vi "make_axes_labels_number_axis.vi"(0 "Merged Array Out":T3(array[cluster]), 1 "View Direction":T1(ring), 2 "Which Axis?":T2(ring)=enum."Z Opposite", 3 "Draw Y?":bool, 5 "from":dbl, 9 "to":dbl, 11 "axis-offset":dbl, 12 "Font Color":u32(colorbox)=4863, 14 "Font Size":dbl min=-1.7976931348623157e+308 max=1.7976931348623157e+308) -> (4 "Scene:New Object":refnum<vi>, 6 "Max Width":dbl)   [LabVIEW 2020, in "3DPC_SurfacePlot.xctl"]
uses:
  <vilib>/Native 3D Graph/xcontrol/3DPC_SurfacePlot.xctl
  <vilib>/Utility/miscctls.llb/LV3DPointTypeDef.ctl
panel:
  in  "Antialiasing":bool
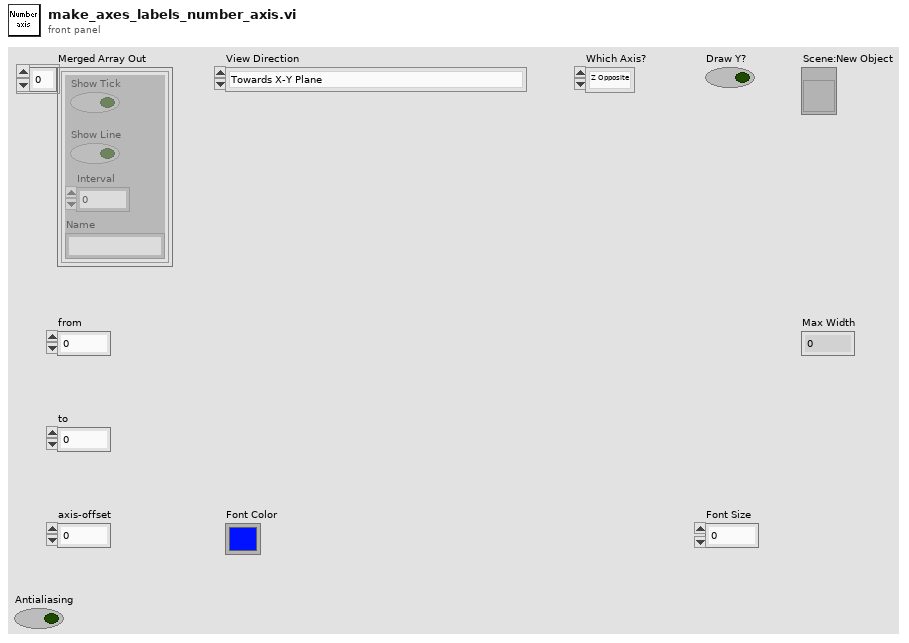
[diagram p1: front panel]
types:
  T1 = enum32{"Towards X-Y Plane", "Towards Y-Z Plane", "Towards X-Z Plane", "User Define"}
  T2 = enum16{"X", "Y", "Z", "X Opposite", "Y Opposite", "Z Opposite"}
  T3 = cluster{"Show Tick":bool, "Show Line":bool, "Interval":sgl, "Name":string}[]
  T4 = typedef "LV3DPointTypeDef.ctl" = cluster{"X":sgl, "Y":sgl, "Z":sgl}
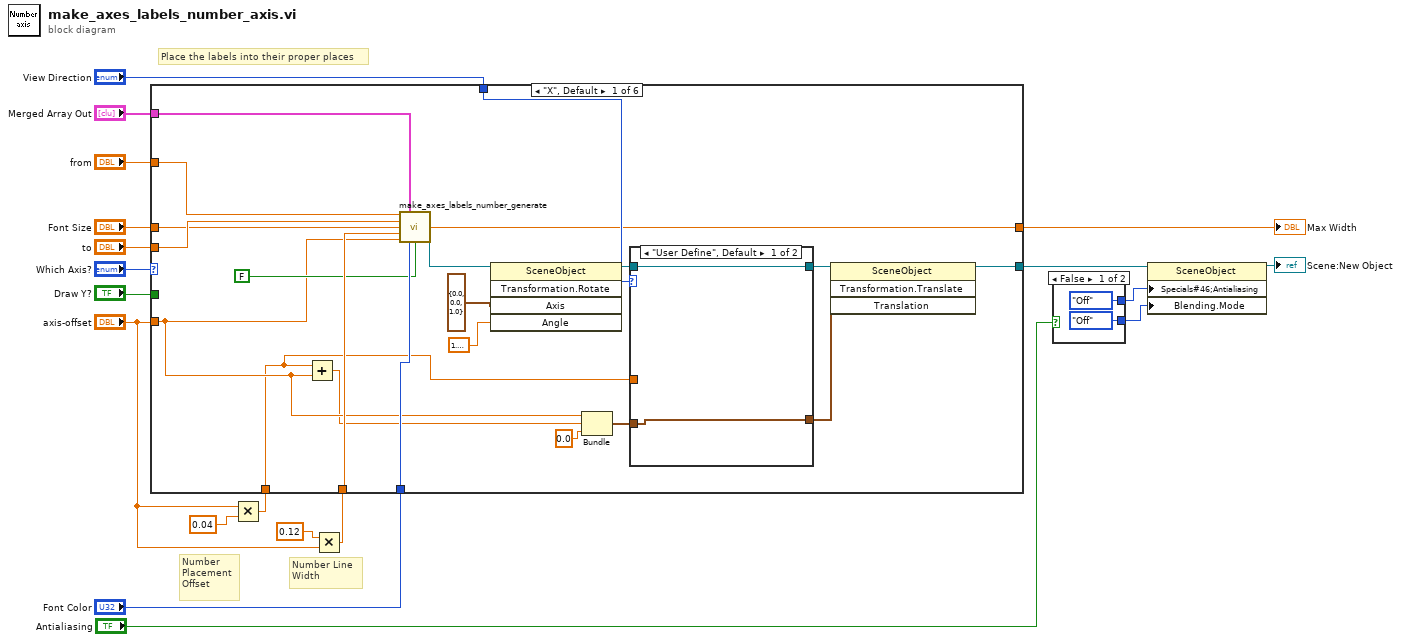
[diagram p0: block diagram]
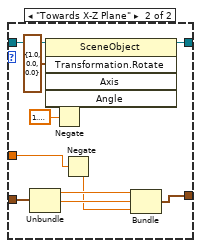
[diagram p2: hidden frame]
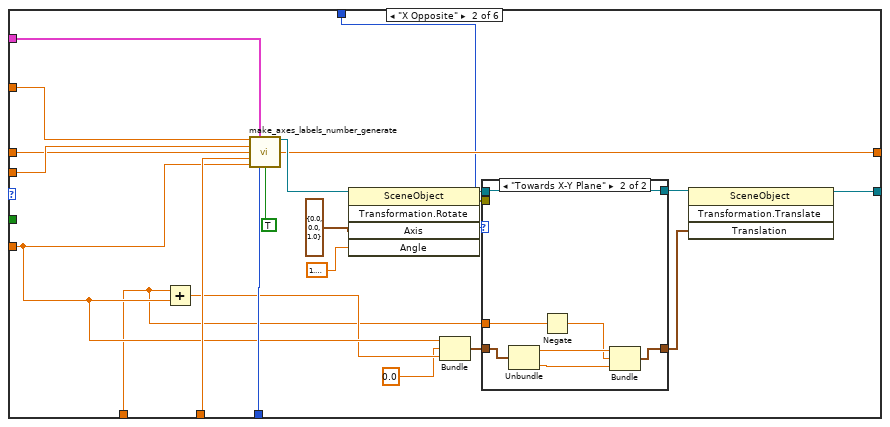
[diagram p3: hidden frame]
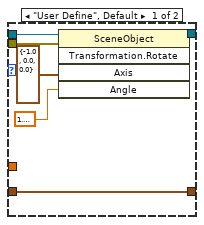
[diagram p4: hidden frame]
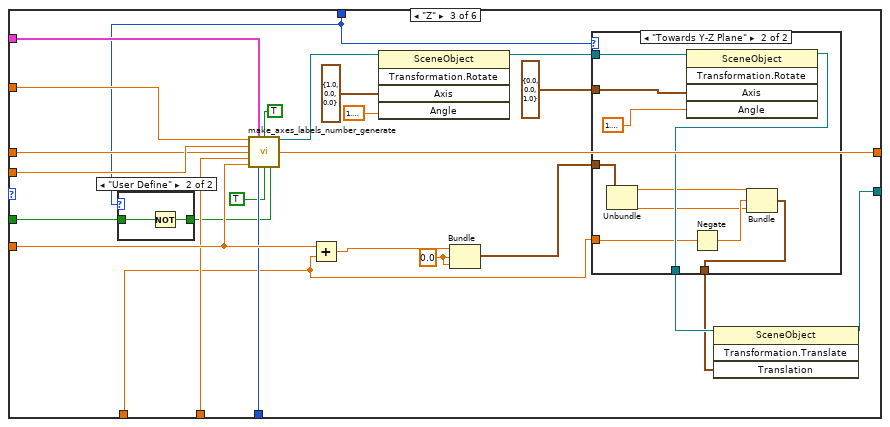
[diagram p5: hidden frame]
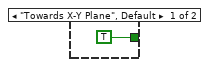
[diagram p6: hidden frame]
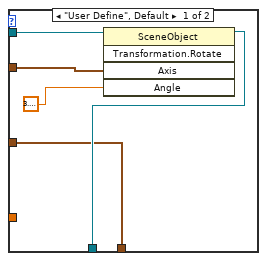
[diagram p7: hidden frame]
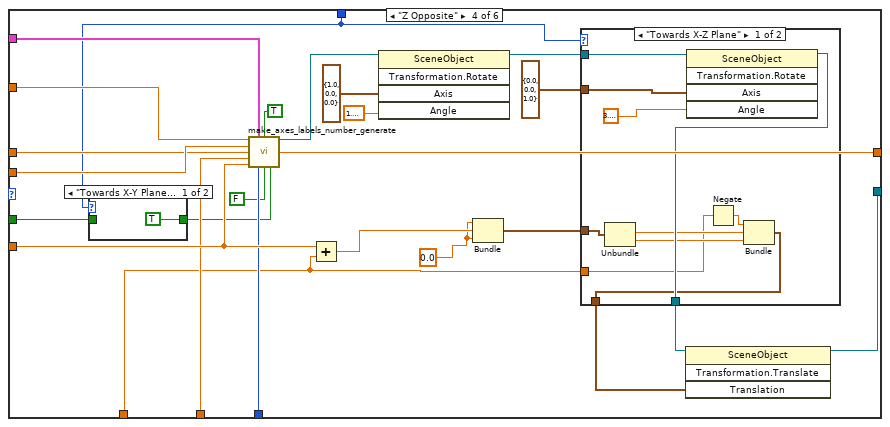
[diagram p8: hidden frame]
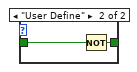
[diagram p9: hidden frame]
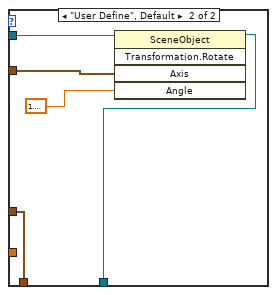
[diagram p10: hidden frame]
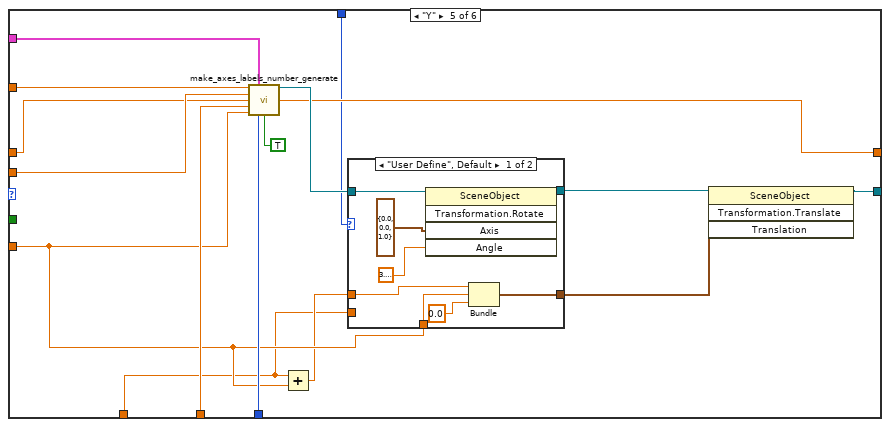
[diagram p11: hidden frame]
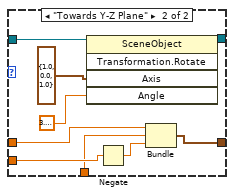
[diagram p12: hidden frame]
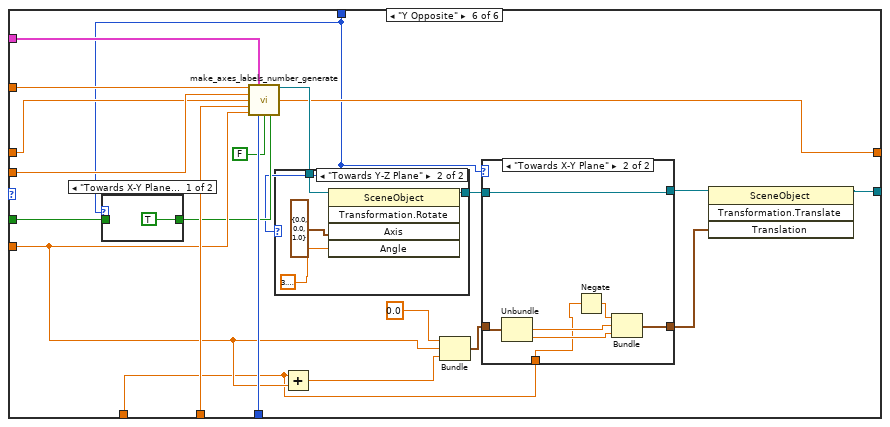
[diagram p13: hidden frame]
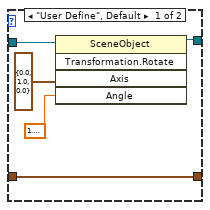
[diagram p14: hidden frame]
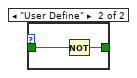
[diagram p15: hidden frame]
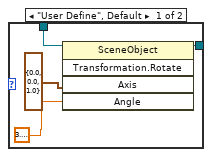
[diagram p16: hidden frame]
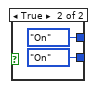
[diagram p17: hidden frame]
diagram:
  # "Place the labels into their proper places"
  # "Number \nPlacement\nOffset"
  # "Number Line\nWidth"
  n1 = Multiply(x="axis-offset", y=0.04 ("x")) -> (x*y=w6:dbl)
  n2 = Multiply(x=0.12 ("width"), y="axis-offset") -> (x*y=w16:dbl)
  n3 = case shown="\"X\", Default" "Which Axis?" {
    tunnel: "from" -> [w39 w74 w100 w143 w189 w227]
    tunnel: "to" -> [w38 w73 w101 w144 w188 w226]
    tunnel: "axis-offset" -> [w26 w61 w106 w149 w178 w216]
    tunnel: [w37 w71 w110 w153 w186 w225] -> w19
    tunnel: w6 -> [w22 w54 w89 w132 w175 w208]
    tunnel: w16 -> [w36 w69 w105 w148 w185 w224]
    tunnel: "Font Color" -> [w35 w68 w104 w147 w184 w223]
    tunnel: [w23 w66 w98 w141 w182 w221] -> w9
    tunnel: "Merged Array Out" -> [w33 w65 w97 w140 w181 w220]
    tunnel: "Draw Y?" -> [_ _ w96 w138 _ w214]
    tunnel: "Font Size" -> [w32 w58 w95 w137 w180 w212]
    tunnel: "View Direction" -> [w27 w57 w94 w136 w179 w211]
    frame "X", Default {
      n4 = Add(x=w22, y=w26) -> (x+y=w20:dbl)
      n5 = call <vilib>:"make_axes_labels_number_generate.vi"("from"=w39, "Merged Array Out"=w33, "to"=w38, "Font Size"=w32, "width"=w36, "height"=w26, "Color Box"=w35, "Right justified"=FALSE) -> ("Scene:New Object"=w40:refnum<vi>, "Max Width"=w23:dbl)  [unwired: 3 in, 3 out]
      n6 = invoke class="SceneObject" method="Transformation.Rotate"(reference=w40, "Axis"=cluster{"X":sgl, "Y":sgl, "Z":sgl} {"X"=0.0, "Y"=0.0, "Z"=1.0}, "Angle"=1.5707963267948966) -> (reference out=w29:refnum<vi>)  [unwired: 2 in, 4 out]
      n7 = Bundle("axis-offset"=w26, w20, "Y"=sgl 0.0) -> (w25:cluster{"axis-offset":dbl, dbl, "Y":sgl})  [unwired: 1 out]
      n8 = case shown="\"User Define\", Default" w27 {
        tunnel: w29 -> [w42 w53]
        tunnel: [w42 w52] -> w28
        tunnel: w25 -> [w41 w43]
        tunnel: [w41 w47] -> w24
        tunnel: w22 -> [_ w45]
        frame "User Define", Default {
        }
        frame "Towards X-Z Plane" {
          n9 = Unbundle(w43) -> ("axis-offset"=w48:dbl, w46:dbl)  [unwired: 1 out]
          n10 = Negate(x=1.5707963267948966) -> (-x=w49:dbl)
          n11 = invoke class="SceneObject" method="Transformation.Rotate"(reference=w53, "Axis"=T4 {"X"=1.0, "Y"=0.0, "Z"=0.0}, "Angle"=w49) -> (reference out=w52:refnum<vi>)  [unwired: 2 in, 4 out]
          n12 = Negate(x=w45) -> (-x=w44:dbl)
          n13 = Bundle("axis-offset"=w48, w46, w44) -> (w47:cluster{"axis-offset":dbl, dbl, dbl})  [unwired: 1 out]
        }
      }
      n14 = invoke class="SceneObject" method="Transformation.Translate"(reference=w28, "Translation"=w24) -> (reference out=w37:refnum<vi>)  [unwired: 2 in, 3 out]
    }
    frame "X Opposite" {
      n15 = Add(x=w54, y=w61) -> (x+y=w60:dbl)
      n16 = call <vilib>:"make_axes_labels_number_generate.vi"("from"=w74, "Merged Array Out"=w65, "to"=w73, "Font Size"=w58, "width"=w69, "height"=w61, "Color Box"=w68, "Right justified"=TRUE) -> ("Scene:New Object"=w75:refnum<vi>, "Max Width"=w66:dbl)  [unwired: 3 in, 3 out]
      n17 = invoke class="SceneObject" method="Transformation.Rotate"(reference=w75, "Axis"=cluster{"X":sgl, "Y":sgl, "Z":sgl} {"X"=0.0, "Y"=0.0, "Z"=1.0}, "Angle"=1.5707963267948966) -> (reference out=w63:refnum<vi>, error out=w64:errorcluster)  [unwired: 2 in, 3 out]
      n18 = Bundle("axis-offset"=w61, "Z"=sgl 0.0, w60) -> (w56:cluster{"axis-offset":dbl, "Z":sgl, dbl})  [unwired: 1 out]
      n19 = case shown="\"Towards X-Y Plane\"" w57 {
        tunnel: w64 -> [w81 _]
        tunnel: w63 -> [w80 w88]
        tunnel: [w79 w88] -> w62
        tunnel: w56 -> [w76 w87]
        tunnel: [w76 w86] -> w55
        tunnel: w54 -> [_ w85]
        frame "User Define", Default {
          n20 = invoke class="SceneObject" method="Transformation.Rotate"(reference=w80, error in=w81, "Axis"=cluster{"X":sgl, "Y":sgl, "Z":sgl} {"X"=-1.0, "Y"=0.0, "Z"=0.0}, "Angle"=1.5707963267948966) -> (reference out=w79:refnum<vi>)  [unwired: 1 in, 4 out]
        }
        frame "Towards X-Y Plane" {
          n21 = Unbundle(w87) -> ("axis-offset"=w83:dbl, w84:dbl)  [unwired: 1 out]
          n22 = Negate(x=w85) -> (-x=w82:dbl)
          n23 = Bundle("axis-offset"=w83, w82, w84) -> (w86:cluster{"axis-offset":dbl, dbl, dbl})  [unwired: 1 out]
        }
      }
      n24 = invoke class="SceneObject" method="Transformation.Translate"(reference=w62, "Translation"=w55) -> (reference out=w71:refnum<vi>)  [unwired: 2 in, 3 out]
    }
    frame "Z" {
      w93 = sgl 0.0 ("Z")
      n25 = case shown="\"User Define\"" w94 {
        tunnel: [TRUE w116] -> w102
        tunnel: w96 -> [_ w115]
        frame "Towards X-Y Plane", Default {
        }
        frame "User Define" {
          n26 = Not(x=w115) -> (.not. x?=w116:bool)
        }
      }
      n27 = call <vilib>:"make_axes_labels_number_generate.vi"("from"=w100, "Merged Array Out"=w97, "Reverse?"=TRUE, "to"=w101, "Font Size"=w95, "width"=w105, "height"=w106, "Color Box"=w104, "Right justified"=TRUE, "Draw Last Label?"=w102) -> ("Scene:New Object"=w113:refnum<vi>, "Max Width"=w98:dbl)  [unwired: 1 in, 3 out]
      n28 = Add(x=w106, y=w89) -> (x+y=w91:dbl)
      n29 = invoke class="SceneObject" method="Transformation.Rotate"(reference=w113, "Axis"=cluster{"X":sgl, "Y":sgl, "Z":sgl} {"X"=1.0, "Y"=0.0, "Z"=0.0}, "Angle"=1.5707963267948966) -> (reference out=w109:refnum<vi>)  [unwired: 2 in, 4 out]
      n30 = Bundle(w91, "Z"=w93, "Z"=w93) -> (w92:cluster{dbl, "Z":sgl, "Z":sgl})  [unwired: 1 out]
      n31 = case shown="\"Towards Y-Z Plane\"" w94 {
        tunnel: w109 -> [w121 w131]
        tunnel: [w120 w130] -> w108
        tunnel: cluster{"X":sgl, "Y":sgl, "Z":sgl} {"X"=0.0, "Y"=0.0, "Z"=1.0} ("Axis") -> [w119 w129]
        tunnel: w92 -> [w117 w126]
        tunnel: w89 -> [_ w124]
        tunnel: [w117 w122] -> w90
        frame "User Define", Default {
          n32 = invoke class="SceneObject" method="Transformation.Rotate"(reference=w121, "Axis"=w119, "Angle"=3.141592653589793) -> (reference out=w120:refnum<vi>)  [unwired: 2 in, 4 out]
        }
        frame "Towards Y-Z Plane" {
          n33 = Unbundle(w126) -> (w125:dbl, "Z"=w123:sgl)  [unwired: 1 out]
          n34 = invoke class="SceneObject" method="Transformation.Rotate"(reference=w131, "Axis"=w129, "Angle"=1.5707963267948966) -> (reference out=w130:refnum<vi>)  [unwired: 2 in, 4 out]
          n35 = Negate(x=w124) -> (-x=w127:dbl)
          n36 = Bundle(w125, w127, "Z"=w123) -> (w122:cluster{dbl, dbl, "Z":sgl})  [unwired: 1 out]
        }
      }
      n37 = invoke class="SceneObject" method="Transformation.Translate"(reference=w108, "Translation"=w90) -> (reference out=w110:refnum<vi>)  [unwired: 2 in, 3 out]
    }
    frame "Z Opposite" {
      w135 = sgl 0.0 ("Z")
      n38 = case shown="\"Towards X-Y Plane\", Default" w136 {
        tunnel: [TRUE w159] -> w145
        tunnel: w138 -> [_ w158]
        frame "Towards X-Y Plane", Default {
        }
        frame "User Define" {
          n39 = Not(x=w158) -> (.not. x?=w159:bool)
        }
      }
      n40 = call <vilib>:"make_axes_labels_number_generate.vi"("from"=w143, "Merged Array Out"=w140, "Reverse?"=TRUE, "to"=w144, "Font Size"=w137, "width"=w148, "height"=w149, "Color Box"=w147, "Right justified"=FALSE, "Draw Last Label?"=w145) -> ("Scene:New Object"=w156:refnum<vi>, "Max Width"=w141:dbl)  [unwired: 1 in, 3 out]
      n41 = Add(x=w149, y=w132) -> (x+y=w139:dbl)
      n42 = invoke class="SceneObject" method="Transformation.Rotate"(reference=w156, "Axis"=cluster{"X":sgl, "Y":sgl, "Z":sgl} {"X"=1.0, "Y"=0.0, "Z"=0.0}, "Angle"=1.5707963267948966) -> (reference out=w152:refnum<vi>)  [unwired: 2 in, 4 out]
      n43 = Bundle("Z"=w135, w139, "Z"=w135) -> (w134:cluster{"Z":sgl, dbl, "Z":sgl})  [unwired: 1 out]
      n44 = case shown="\"Towards X-Z Plane\"" w136 {
        tunnel: w152 -> [w169 w174]
        tunnel: [w168 w173] -> w151
        tunnel: cluster{"X":sgl, "Y":sgl, "Z":sgl} {"X"=0.0, "Y"=0.0, "Z"=1.0} ("Axis") -> [w167 w172]
        tunnel: w134 -> [w165 w170]
        tunnel: [w163 w170] -> w133
        tunnel: w132 -> [w161 _]
        frame "Towards X-Z Plane" {
          n45 = Unbundle(w165) -> (w164:dbl, "Z"=w162:sgl)  [unwired: 1 out]
          n46 = invoke class="SceneObject" method="Transformation.Rotate"(reference=w169, "Axis"=w167, "Angle"=3.141592653589793) -> (reference out=w168:refnum<vi>)  [unwired: 2 in, 4 out]
          n47 = Negate(x=w161) -> (-x=w160:dbl)
          n48 = Bundle(w160, w164, "Z"=w162) -> (w163:cluster{dbl, dbl, "Z":sgl})  [unwired: 1 out]
        }
        frame "User Define", Default {
          n49 = invoke class="SceneObject" method="Transformation.Rotate"(reference=w174, "Axis"=w172, "Angle"=1.5707963267948966) -> (reference out=w173:refnum<vi>)  [unwired: 2 in, 4 out]
        }
      }
      n50 = invoke class="SceneObject" method="Transformation.Translate"(reference=w151, "Translation"=w133) -> (reference out=w153:refnum<vi>)  [unwired: 2 in, 3 out]
    }
    frame "Y" {
      n51 = call <vilib>:"make_axes_labels_number_generate.vi"("from"=w189, "Merged Array Out"=w181, "to"=w188, "Font Size"=w180, "width"=w185, "height"=w178, "Color Box"=w184, "Right justified"=TRUE) -> ("Scene:New Object"=w190:refnum<vi>, "Max Width"=w182:dbl)  [unwired: 3 in, 3 out]
      n52 = Add(x=w175, y=w178) -> (x+y=w177:dbl)
      n53 = case shown="\"User Define\", Default" w179 {
        tunnel: w190 -> [w198 w207]
        tunnel: [w196 w205] -> w187
        tunnel: w178 -> [w192 w200]
        tunnel: w177 -> [w191 w199]
        tunnel: [w193 w201] -> w176
        tunnel: w175 -> [_ w203]
        frame "User Define", Default {
          n54 = invoke class="SceneObject" method="Transformation.Rotate"(reference=w198, "Axis"=cluster{"X":sgl, "Y":sgl, "Z":sgl} {"X"=0.0, "Y"=0.0, "Z"=1.0}, "Angle"=3.141592653589793) -> (reference out=w196:refnum<vi>)  [unwired: 2 in, 4 out]
          n55 = Bundle(w191, "axis-offset"=w192, "width"=0.0) -> (w193:cluster{dbl, "axis-offset":dbl, "width":dbl})  [unwired: 1 out]
        }
        frame "Towards Y-Z Plane" {
          n56 = invoke class="SceneObject" method="Transformation.Rotate"(reference=w207, "Axis"=cluster{"X":sgl, "Y":sgl, "Z":sgl} {"X"=1.0, "Y"=0.0, "Z"=1.0}, "Angle"=3.141592653589793) -> (reference out=w205:refnum<vi>)  [unwired: 2 in, 4 out]
          n57 = Negate(x=w203) -> (-x=w202:dbl)
          n58 = Bundle(w199, "axis-offset"=w200, w202) -> (w201:cluster{dbl, "axis-offset":dbl, dbl})  [unwired: 1 out]
        }
      }
      n59 = invoke class="SceneObject" method="Transformation.Translate"(reference=w187, "Translation"=w176) -> (reference out=w186:refnum<vi>)  [unwired: 2 in, 3 out]
    }
    frame "Y Opposite" {
      n60 = case shown="\"Towards X-Y Plane\", Default" w211 {
        tunnel: w214 -> [_ w243]
        tunnel: [TRUE w242] -> w213
        frame "Towards X-Y Plane", Default {
        }
        frame "User Define" {
          n61 = Not(x=w243) -> (.not. x?=w242:bool)
        }
      }
      n62 = call <vilib>:"make_axes_labels_number_generate.vi"("from"=w227, "Merged Array Out"=w220, "to"=w226, "Font Size"=w212, "width"=w224, "height"=w216, "Color Box"=w223, "Right justified"=FALSE, "Draw Last Label?"=w213) -> ("Scene:New Object"=w228:refnum<vi>, "Max Width"=w221:dbl)  [unwired: 2 in, 3 out]
      n63 = case shown="\"Towards Y-Z Plane\"" w211 {
        tunnel: w228 -> [w247 w251]
        tunnel: [w245 w249] -> w219
        frame "User Define", Default {
          n64 = invoke class="SceneObject" method="Transformation.Rotate"(reference=w247, "Axis"=cluster{"X":sgl, "Y":sgl, "Z":sgl} {"X"=0.0, "Y"=0.0, "Z"=1.0}, "Angle"=3.141592653589793) -> (reference out=w245:refnum<vi>)  [unwired: 2 in, 4 out]
        }
        frame "Towards Y-Z Plane" {
          n65 = invoke class="SceneObject" method="Transformation.Rotate"(reference=w251, "Axis"=cluster{"X":sgl, "Y":sgl, "Z":sgl} {"X"=0.0, "Y"=0.0, "Z"=1.0}, "Angle"=3.141592653589793) -> (reference out=w249:refnum<vi>)  [unwired: 2 in, 4 out]
        }
      }
      n66 = Add(x=w208, y=w216) -> (x+y=w215:dbl)
      n67 = Bundle("Z"=sgl 0.0, "axis-offset"=w216, w215) -> (w210:cluster{"Z":sgl, "axis-offset":dbl, dbl})  [unwired: 1 out]
      n68 = case shown="\"Towards X-Y Plane\"" w211 {
        tunnel: w219 -> [w233 w240]
        tunnel: [w232 w240] -> w218
        tunnel: w210 -> [w229 w239]
        tunnel: [w229 w238] -> w209
        tunnel: w208 -> [_ w235]
        frame "User Define", Default {
          n69 = invoke class="SceneObject" method="Transformation.Rotate"(reference=w233, "Axis"=cluster{"X":sgl, "Y":sgl, "Z":sgl} {"X"=0.0, "Y"=1.0, "Z"=0.0}, "Angle"=1.5707963267948966) -> (reference out=w232:refnum<vi>)  [unwired: 2 in, 4 out]
        }
        frame "Towards X-Y Plane" {
          n70 = Unbundle(w239) -> ("axis-offset"=w237:dbl, w236:dbl)  [unwired: 1 out]
          n71 = Negate(x=w235) -> (-x=w234:dbl)
          n72 = Bundle(w234, "axis-offset"=w237, w236) -> (w238:cluster{dbl, "axis-offset":dbl, dbl})  [unwired: 1 out]
        }
      }
      n73 = invoke class="SceneObject" method="Transformation.Translate"(reference=w218, "Translation"=w209) -> (reference out=w225:refnum<vi>)  [unwired: 2 in, 3 out]
    }
  }
  "Max Width" <- w9
  n74 = case shown="False" "Antialiasing" {
    tunnel: [enum16{"Inherit Value", "Off", "On"}."Off" ("Blending:Mode") enum16{"Inherit Value", "Off", "On"}."On" ("Blending:Mode")] -> w12
    tunnel: [enum16{"Inherit Value", "Off", "On"}."Off" ("Specials:Antialiasing") enum16{"Inherit Value", "Off", "On"}."On" ("Specials:Antialiasing")] -> w11
    frame False {
    }
    frame True {
    }
  }
  n75 = property class="SceneObject"(reference=w19, "Specials#46;Antialiasing"=w12, "Blending.Mode"=w11) -> (reference out=→"Scene:New Object":refnum<vi>)  [unwired: 1 in, 1 out]
